vi "refract.vi"(9 "RefractInd":dbl, 10 "N":dbl[](array[numeric]), 11 "I":dbl[](array[numeric])) -> (3 "Refract":dbl[](array[numeric]))   [LabVIEW 2015]
uses:
  <vilib>/Analysis/baseanly.llb/Real Dot Product.vi
  <vilib>/Analysis/NI_AALBase.lvlib
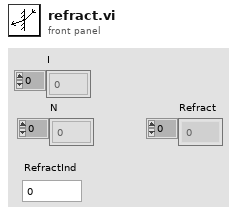
[diagram p1: front panel]
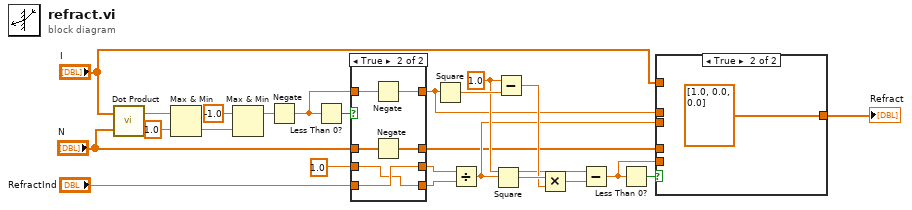
[diagram p0: block diagram]
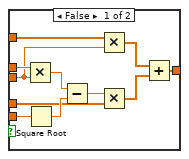
[diagram p2: hidden frame]
diagram:
  w8 = 1.0 ("x")
  n1 = call-poly <vilib>:"Dot Product.vi"("Y Vector"="N", "X Vector"="I") -> ("X * Y"=w24:dbl)  [unwired: 1 out]
  n2 = Max & Min(x=w24, y=1.0) -> (min(x,y)=w22:dbl)  [unwired: 1 out]
  n3 = Max & Min(x=-1.0, y=w22) -> (max(x,y)=w20:dbl)  [unwired: 1 out]
  n4 = Negate(x=w20) -> (-x=w18:dbl)
  n5 = Less Than 0?(x=w18) -> (x < 0?=w19:bool)
  n6 = case shown="True" w19 {
    tunnel: w18 -> [w25 w34]
    tunnel: [w25 w33] -> w3
    tunnel: "RefractInd" -> [w28 w32]
    tunnel: "N" -> [w26 w31]
    tunnel: [w27 w32] -> w14
    tunnel: [w28 w29] -> w13
    tunnel: [w26 w30] -> w2
    tunnel: 1.0 -> [w27 w29]
    frame False {
    }
    frame True {
      n7 = Negate(x=w34) -> (-x=w33:dbl)
      n8 = Negate(x=w31) -> (-x=w30:dbl[])
    }
  }
  n9 = Square(x=w3) -> (x^2=w12:dbl)
  n10 = Divide(x=w14, y=w13) -> (x/y=w4:dbl)
  n11 = Square(x=w4) -> (x^2=w11:dbl)
  n12 = Subtract(x=w8, y=w12) -> (x-y=w10:dbl)
  n13 = Multiply(x=w11, y=w10) -> (x*y=w9:dbl)
  n14 = Subtract(x=w8, y=w9) -> (x-y=w5:dbl)
  n15 = Less Than 0?(x=w5) -> (x < 0?=w7:bool)
  n16 = case shown="True" w7 {
    tunnel: [w35 dbl[] [1.0, 0.0, 0.0] ("Refract")] -> w6
    tunnel: w5 -> [w44 _]
    tunnel: w4 -> [w39 _]
    tunnel: w3 -> [w45 _]
    tunnel: w2 -> [w42 _]
    tunnel: "I" -> [w38 _]
    frame False {
      n17 = Multiply(x=w45, y=w39) -> (x*y=w40:dbl)
      n18 = Square Root(x=w44) -> (sqrt(x)=w43:dbl)
      n19 = Subtract(x=w40, y=w43) -> (x-y=w41:dbl)
      n20 = Multiply(x=w38, y=w39) -> (x*y=w37:dbl[])
      n21 = Multiply(x=w41, y=w42) -> (x*y=w36:dbl[])
      n22 = Add(x=w37, y=w36) -> (x+y=w35:dbl[])
    }
    frame True {
    }
  }
  "Refract" <- w6
